vi "ZeroMQ_SUBGS.vi"() -> ()   [LabVIEW 2018]
uses:
  <vilib>/addons/zeromq/socket_type.ctl
  <vilib>/addons/zeromq/socket_options.ctl
  <vilib>/addons/zeromq/zeromq.lvlib
  <vilib>/addons/zeromq/zmq_socket.lvclass
  <vilib>/addons/zeromq/zmq_context.lvclass
panel:
  out "error out 5":errorcluster
  in  "stop 4":bool
  out "command 2":string
  out "reply":string
  out "message 2":string
  out "error out 4":errorcluster
  out "error out 3":errorcluster
  out "error out 2":errorcluster
  out "message":string
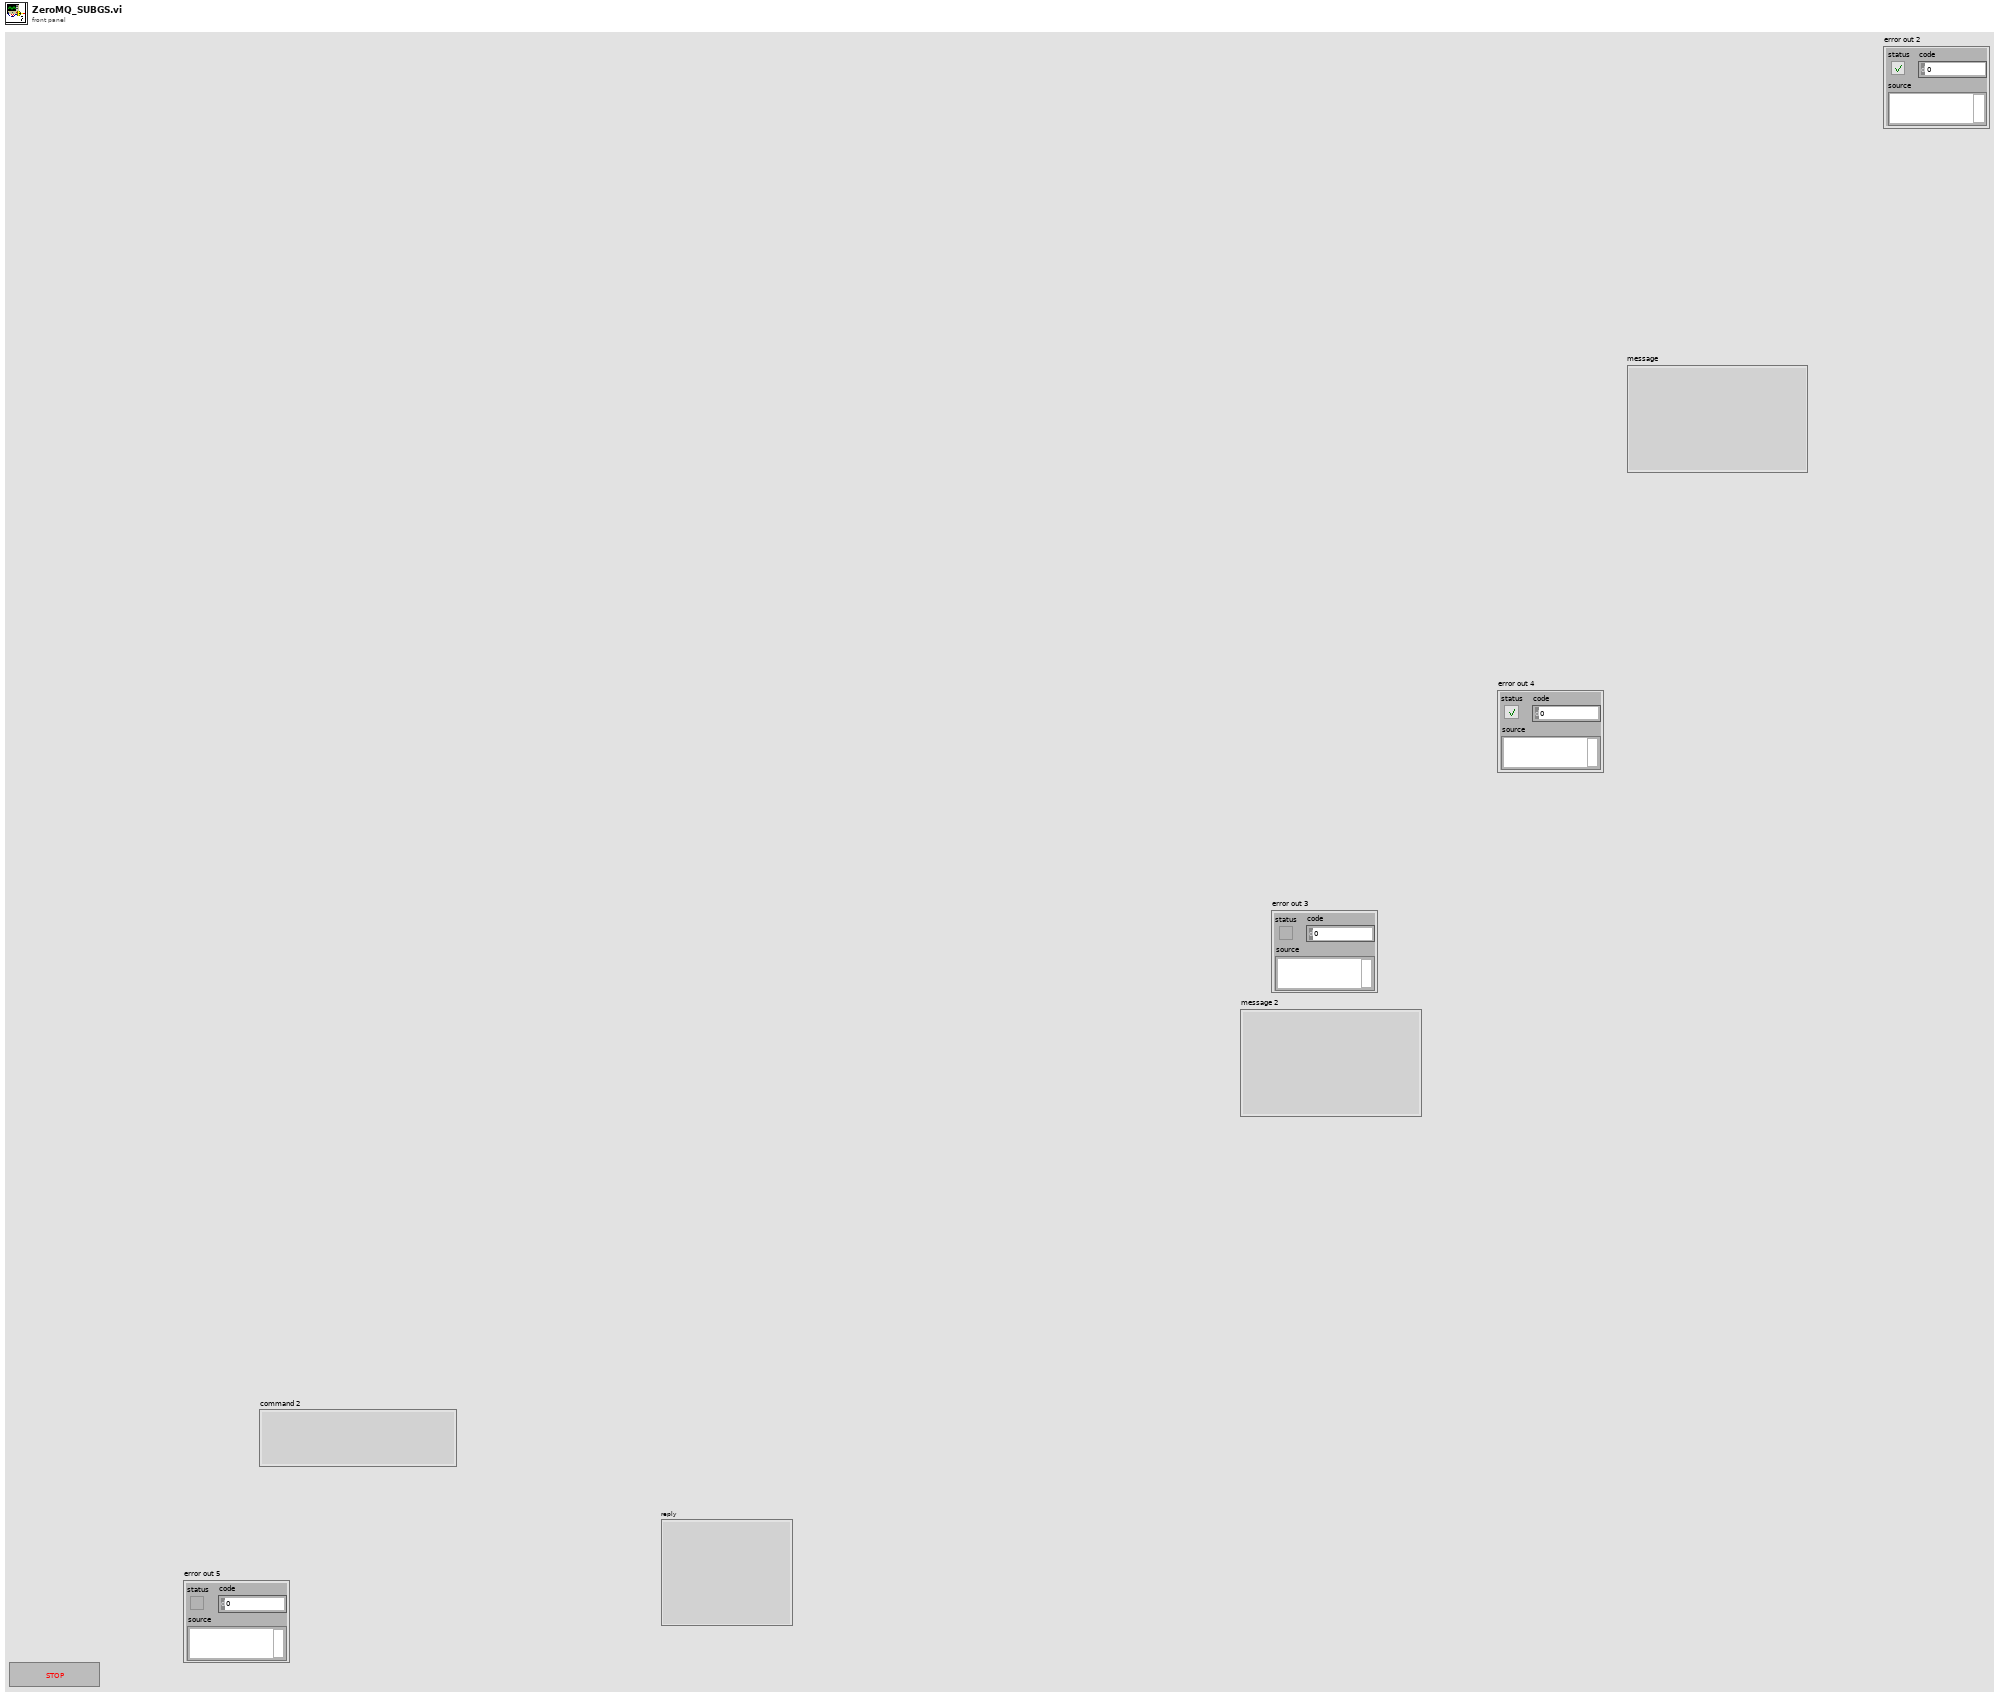
[diagram p1: front panel]
types:
  T1 = typedef "zeromq.lvlib/socket_options.ctl" = enum8{"NONE", "ZMQ_HWM", "<2>", "ZMQ_SWAP", "ZMQ_AFFINITY", "ZMQ_ROUTING_ID", "ZMQ_SUBSCRIBE", "ZMQ_UNSUBSCRIBE", "ZMQ_RATE", "ZMQ_RECOVERY_IVL", "ZMQ_MCAST_LOOP", "ZMQ_SNDBUF", "ZMQ_RCVBUF", "ZMQ_RCVMORE", "ZMQ_FD", "ZMQ_EVENTS", "ZMQ_TYPE", "ZMQ_LINGER", "ZMQ_RECONNECT_IVL", "ZMQ_BACKLOG", "ZMQ_RECOVERY_IVL_MSEC", "ZMQ_RECONNECT_IVL_MAX", "ZMQ_MAXMSGSIZE", "ZMQ_SNDHWM", "ZMQ_RCVHWM", "ZMQ_MULTICAST_HOPS", "<26>", "ZMQ_RCVTIMEO", "ZMQ_SNDTIMEO", "<29>", "<30>", "ZMQ_IPV4ONLY", "ZMQ_LAST_ENDPOINT", "ZMQ_ROUTER_MANDATORY", "ZMQ_TCP_KEEPALIVE", "ZMQ_TCP_KEEPALIVE_CNT", "ZMQ_TCP_KEEPALIVE_IDLE", "ZMQ_TCP_KEEPALIVE_INTVL", "ZMQ_TCP_ACCEPT_FILTER", "ZMQ_IMMEDIATE", "ZMQ_XPUB_VERBOSE", "ZMQ_ROUTER_RAW", "ZMQ_IPV6", "ZMQ_MECHANISM", "ZMQ_PLAIN_SERVER", "ZMQ_PLAIN_USERNAME", "ZMQ_PLAIN_PASSWORD", "ZMQ_CURVE_SERVER", "ZMQ_CURVE_PUBLICKEY", "ZMQ_CURVE_SECRETKEY", "ZMQ_CURVE_SERVERKEY", "ZMQ_PROBE_ROUTER", "ZMQ_REQ_CORRELATE", "ZMQ_REQ_RELAXED", "ZMQ_CONFLATE", "ZMQ_ZAP_DOMAIN", "ZMQ_ROUTER_HANDOVER", "ZMQ_TOS", "ZMQ_IPC_FILTER_PID", "ZMQ_IPC_FILTER_UID", "ZMQ_IPC_FILTER_GID", "ZMQ_CONNECT_ROUTING_ID", "ZMQ_GSSAPI_SERVER", "ZMQ_GSSAPI_PRINCIPAL", "ZMQ_GSSAPI_SERVICE_PRINCIPAL", "ZMQ_GSSAPI_PLAINTEXT", "ZMQ_HANDSHAKE_IVL", "<67>", "ZMQ_SOCKS_PROXY", "ZMQ_XPUB_NODROP", "ZMQ_BLOCKY", "ZMQ_XPUB_MANUAL", "ZMQ_XPUB_WELCOME_MSG", "ZMQ_STREAM_NOTIFY", "ZMQ_INVERT_MATCHING", "ZMQ_HEARTBEAT_IVL", "ZMQ_HEARTBEAT_TTL", "ZMQ_HEARTBEAT_TIMEOUT", "ZMQ_XPUB_VERBOSER", "ZMQ_CONNECT_TIMEOUT", "ZMQ_TCP_MAXRT", "ZMQ_THREAD_SAFE", "<82>", "<83>", "ZMQ_MULTICAST_MAXTPDU", "ZMQ_VMCI_BUFFER_SIZE", "ZMQ_VMCI_BUFFER_MIN_SIZE", "ZMQ_VMCI_BUFFER_MAX_SIZE", "ZMQ_VMCI_CONNECT_TIMEOUT", "ZMQ_USE_FD", "ZMQ_GSSAPI_PRINCIPAL_NAMETYPE", "ZMQ_GSSAPI_SERVICE_PRINCIPAL_NAMETYPE", "ZMQ_BINDTODEVICE", "ZMQ_ZAP_ENFORCE_DOMAIN", "ZMQ_LOOPBACK_FASTPATH", "ZMQ_METADATA", "ZMQ_MULTICAST_LOOP", "ZMQ_ROUTER_NOTIFY"}
  T2 = typedef "zeromq.lvlib/socket_type.ctl" = enum8{"ZMQ_PAIR", "ZMQ_PUB", "ZMQ_SUB", "ZMQ_REQ", "ZMQ_REP", "ZMQ_DEALER", "ZMQ_ROUTER", "ZMQ_PULL", "ZMQ_PUSH", "ZMQ_XPUB", "ZMQ_XSUB", "ZMQ_STREAM", "ZMQ_SERVER", "ZMQ_CLIENT", "ZMQ_RADIO", "ZMQ_DISH", "ZMQ_GATHER", "ZMQ_SCATTER", "ZMQ_DGRAM"}
  T3 = cluster{"ID":u32, "Address":string, "Service Name 1":string, "Service Name 2":string, "queue TX":refnum<queue>, "queue RX":refnum<queue>, "Port 1":u32, "Port 2":u32}
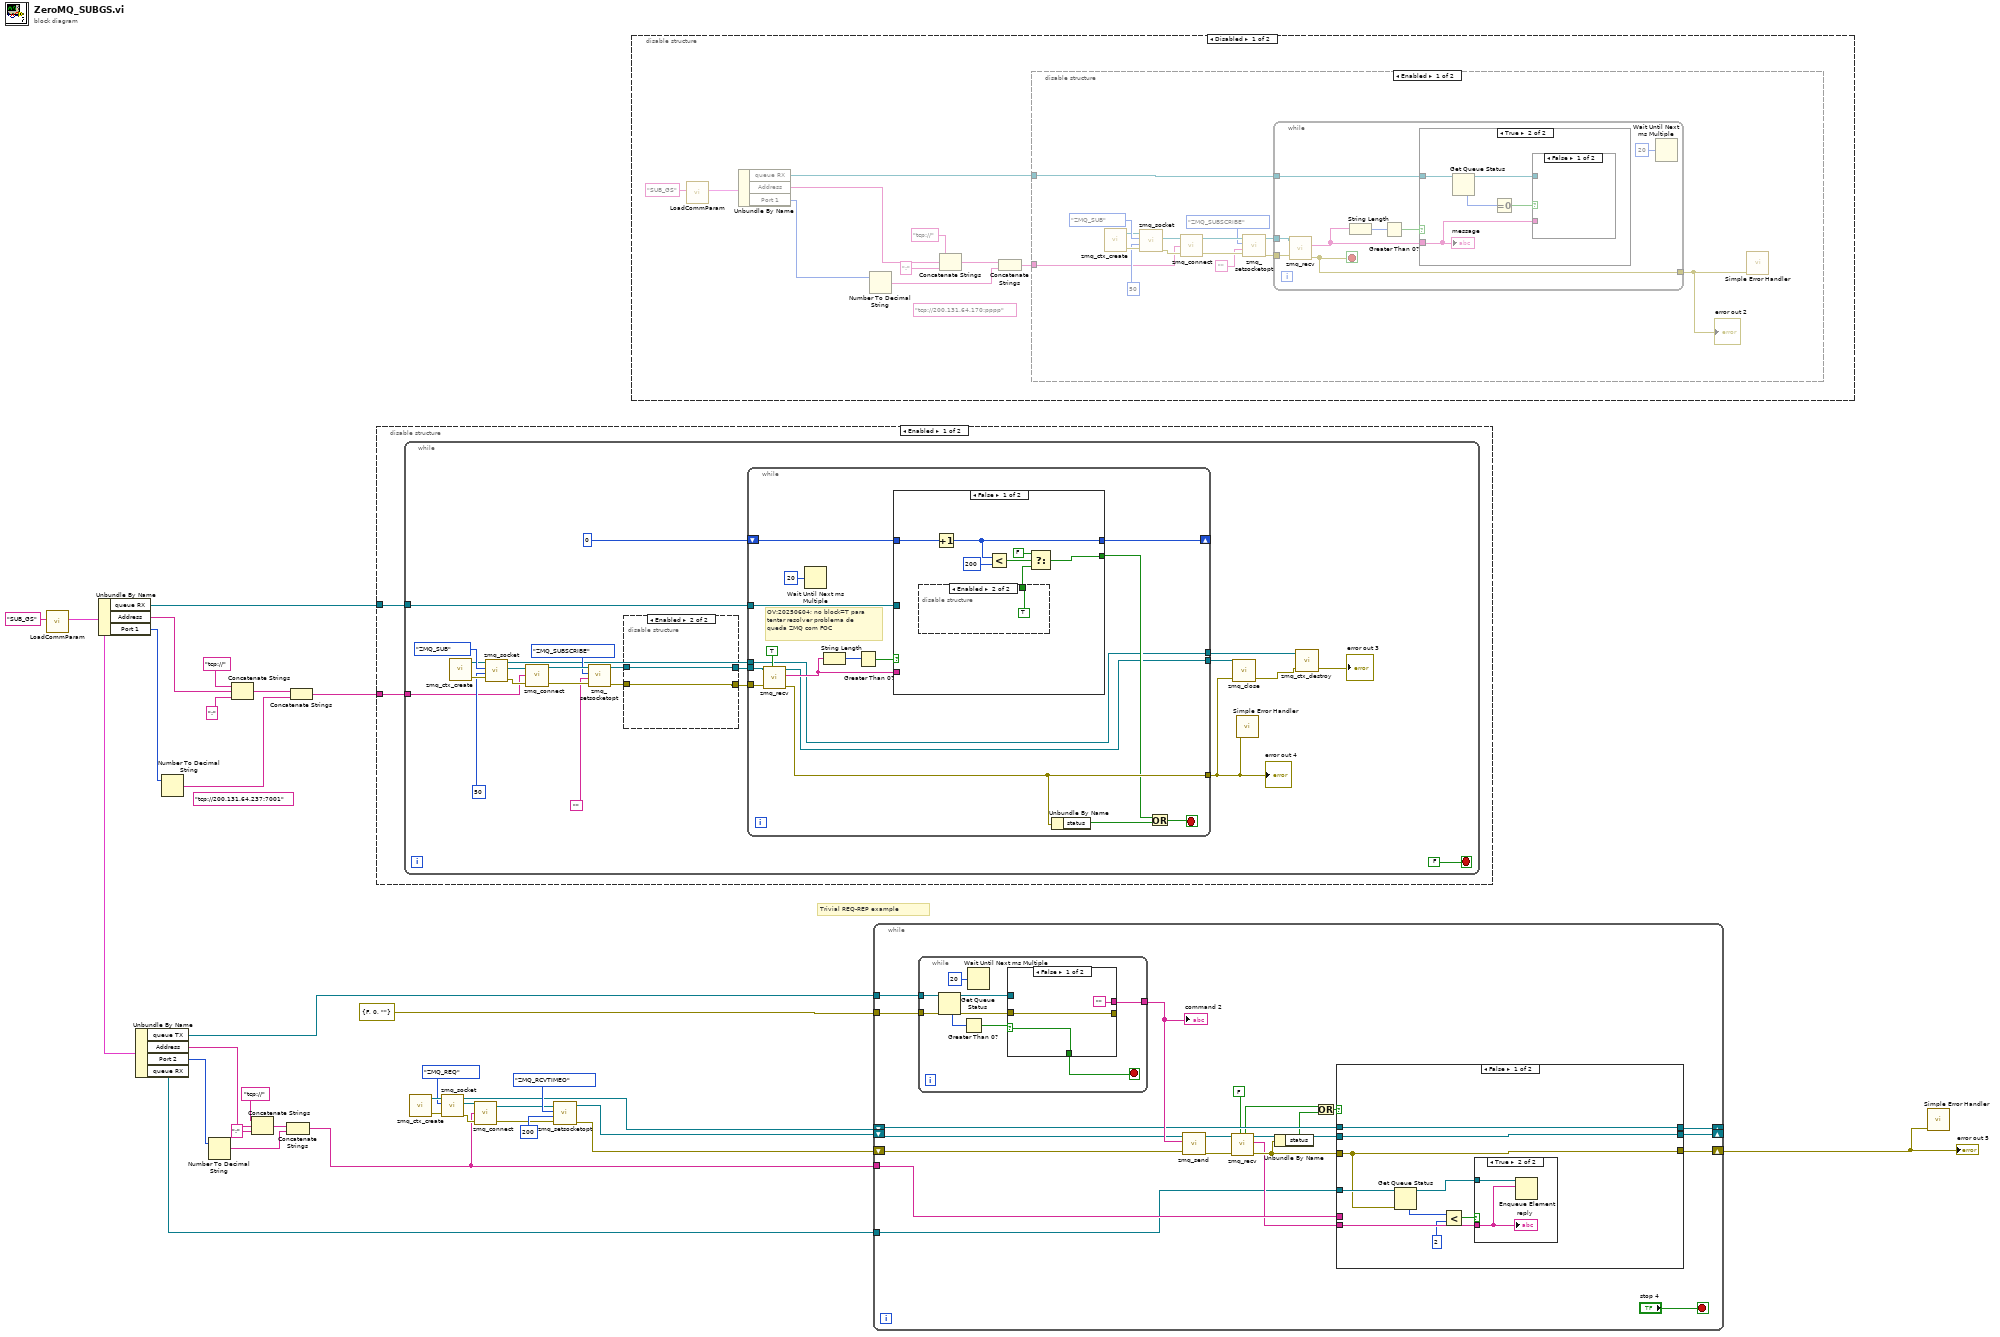
[diagram p0: block diagram]
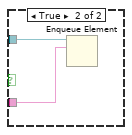
[diagram p3: hidden frame]
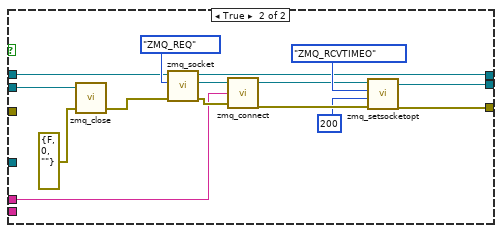
[diagram p7: hidden frame]
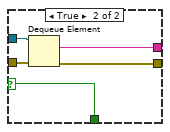
[diagram p8: hidden frame]
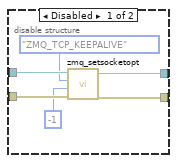
[diagram p9: hidden frame]
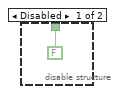
[diagram p10: hidden frame]
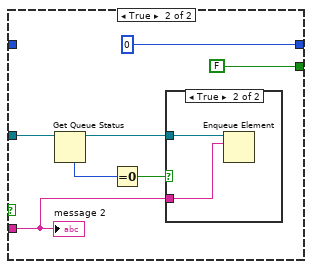
[diagram p11: hidden frame]
diagram:
  (unwired) "tcp://200.131.64.237:7001" ("endpoint")
  # "Trivial REQ-REP example"
  n1 = call "LoadCommParam.vi"("section name"="SUB_GS") -> ("output cluster"=w1:T3)  [unwired: 10 in]
  n2 = Unbundle By Name(w1) -> ("queue RX"=w25:refnum<queue>, "Address"=w32:string, "Port 1"=w31:u32)
  n3 = Unbundle By Name(w1) -> ("queue TX"=w16:refnum<queue>, "Address"=w18:string, "Port 2"=w17:u32, "queue RX"=w2:refnum<queue>)
  n4 = Number To Decimal String(number=w31) -> (decimal integer string=w30:string)  [unwired: 1 in]
  n5 = Number To Decimal String(number=w17) -> (decimal integer string=w22:string)  [unwired: 1 in]
  n6 = Concatenate Strings("tcp://" ("string"), w32, ":" ("string")) -> (w29:string)
  n7 = Concatenate Strings("tcp://" ("string"), w18, ":" ("string")) -> (w21:string)
  n8 = Concatenate Strings(w21, w22) -> (w10:string)
  n9 = Concatenate Strings(w29, w30) -> (w26:string)
  n10 = disable-structure shown="Enabled" {
    disable-tunnel: w25 -> [w35 _]
    disable-tunnel: w26 -> [w34 _]
    frame Enabled {
      n11 = while {
        tunnel: w35 -> [w50]
        tunnel: w34 -> [w49]
        stop <- FALSE stop-if-true
        n12 = call <vilib>:"zmq_ctx_create.vi"() -> ("error out"=w58:errorcluster, "context out"=w52:refnum<class "zmq_context.lvclass">)  [unwired: 4 in]
        n13 = call <vilib>:"zmq_socket.vi"("error in"=w58, "linger (ms)"=50, "socket type"=socket_type."ZMQ_SUB", "context in"=w52) -> ("error out"=w57:errorcluster, "socket out"=w53:refnum<class "zmq_socket.lvclass">, "context out"=w41:refnum<class "zmq_context.lvclass">)  [unwired: 1 in]
        n14 = call <vilib>:"zmq_connect.vi"("error in"=w57, "endpoint"=w49, "socket in"=w53) -> ("error out"=w55:errorcluster, "socket out"=w56:refnum<class "zmq_socket.lvclass">)  [unwired: 1 in]
        n15 = call <vilib>:"zmq_setsocketopt.vi"("error in"=w55, "value"="", "option"=socket_options."ZMQ_SUBSCRIBE", "socket in"=w56) -> ("error out"=w44:errorcluster, "socket out"=w46:refnum<class "zmq_socket.lvclass">)  [unwired: 2 in]
        n16 = disable-structure shown="Enabled" {
          disable-tunnel: w46 -> [w65 w67]
          disable-tunnel: [w64 w67] -> w45
          disable-tunnel: w44 -> [w63 w66]
          disable-tunnel: [w62 w66] -> w43
          frame Disabled {
            n17 = call <vilib>:"zmq_setsocketopt.vi"("error in"=w63, "value"=-1, "option"=socket_options."ZMQ_TCP_KEEPALIVE", "socket in"=w65) -> ("error out"=w62:errorcluster, "socket out"=w64:refnum<class "zmq_socket.lvclass">)  [unwired: 2 in]
          }
          frame Enabled {
          }
        }
        n18 = while {
          tunnel: w45 -> [w82]
          tunnel: w43 -> [w83]
          tunnel: [w73] -> w38
          tunnel: w50 -> [w79]
          shift-right: [w74] -> _
          shift-left: 0 -> [w75]
          tunnel: [w69] -> w40
          tunnel: w41 -> [w68]
          tunnel: [w68] -> w39
          stop <- w70 stop-if-true
          # "OV:20250604; no block=T para\ntentar resolver problema de\nqueda ZMQ com FOC"
          n19 = call <vilib>:"zmq_recv.vi"("no block? (F)"=TRUE, "error in"=w83, "socket in"=w82) -> ("error out"=w73:errorcluster, "data"=w78:string, "socket out"=w69:refnum<class "zmq_socket.lvclass">)  [unwired: 2 in, 2 out]
          n20 = Wait Until Next ms Multiple(millisecond multiple=u32 20) -> ()  [unwired: 1 out]
          n21 = String Length(string=w78) -> (length=w81:i32)
          n22 = Greater Than 0?(x=w81) -> (x > 0?=w80:bool)
          n23 = case shown="False" w80 {
            tunnel: w79 -> [_ w98]
            tunnel: w78 -> [_ w95]
            tunnel: w75 -> [w90 _]
            tunnel: [w89 0] -> w74
            tunnel: [w86 FALSE] -> w71
            frame False {
              n24 = disable-structure shown="Enabled" {
                disable-tunnel: [FALSE ("f") TRUE] -> w84
                frame Disabled {
                }
                frame Enabled {
                }
              }
              n25 = Increment(x=w90) -> (x+1=w89:i32)
              n26 = Less?(x=w89, y=200) -> (x < y?=w87:bool)
              n27 = Select(t=FALSE, s=w87, f=w84) -> (s? t:f=w86:bool)
            }
            frame True {
              n28 = Get Queue Status(queue=w98) -> (queue out=w96:refnum<queue>, # elements in queue=w99:i32)  [unwired: 2 in, 6 out]
              n29 = Equal To 0?(x=w99) -> (x = 0?=w97:bool)
              n30 = case shown="True" w97 {
                tunnel: w96 -> [_ w101]
                tunnel: w95 -> [_ w100]
                frame False {
                }
                frame True {
                  n31 = Enqueue Element(queue=w101, element=w100) -> ()  [unwired: 2 in, 3 out]
                }
              }
              "message 2" <- w95
            }
          }
          n32 = Unbundle By Name(w73) -> ("status"=w72:bool)
          n33 = Or(x=w71, y=w72) -> (x .or. y?=w70:bool)
        }
        "error out 4" <- w38
        n34 = call <vilib>:"zmq_close.vi"("error in"=w38, "socket"=w40) -> ("error out"=w37:errorcluster)  [unwired: 3 in]
        n35 = call <vilib>:"Simple Error Handler.vi"("error in (no error)"=w38) -> ()  [unwired: 4 in, 5 out]
        n36 = call <vilib>:"zmq_ctx_destroy.vi"("error in"=w37, "context in"=w39) -> ("error out"=→"error out 3":errorcluster)  [unwired: 3 in]
      }
    }
    frame Disabled {
    }
  }
  n37 = call <vilib>:"zmq_ctx_create.vi"() -> ("error out"=w15:errorcluster, "context out"=w12:refnum<class "zmq_context.lvclass">)  [unwired: 4 in]
  n38 = call <vilib>:"zmq_socket.vi"("error in"=w15, "socket type"=socket_type."ZMQ_REQ", "context in"=w12) -> ("error out"=w13:errorcluster, "socket out"=w14:refnum<class "zmq_socket.lvclass">, "context out"=w5:refnum<class "zmq_context.lvclass">)  [unwired: 2 in]
  n39 = call <vilib>:"zmq_connect.vi"("error in"=w13, "endpoint"=w10, "socket in"=w14) -> ("error out"=w6:errorcluster, "socket out"=w7:refnum<class "zmq_socket.lvclass">)  [unwired: 1 in]
  n40 = call <vilib>:"zmq_setsocketopt.vi"("error in"=w6, "value"=200 ("max queue size (-1, unlimited)"), "option"=socket_options."ZMQ_RCVTIMEO", "socket in"=w7) -> ("error out"=w3:errorcluster, "socket out"=w4:refnum<class "zmq_socket.lvclass">)  [unwired: 2 in]
  n41 = disable-structure shown="Disabled" {
    frame Disabled {
      (unwired) "tcp://200.131.64.170:pppp" ("endpoint")
      n42 = call "LoadCommParam.vi"("section name"="SUB_GS") -> ("output cluster"=w102:T3)  [unwired: 10 in]
      n43 = Unbundle By Name(w102) -> ("queue RX"=w103:refnum<queue>, "Address"=w110:string, "Port 1"=w109:u32)
      n44 = Number To Decimal String(number=w109) -> (decimal integer string=w108:string)  [unwired: 1 in]
      n45 = Concatenate Strings("tcp://" ("string"), w110, ":" ("string")) -> (w107:string)
      n46 = Concatenate Strings(w107, w108) -> (w104:string)
      n47 = disable-structure shown="Enabled" {
        disable-tunnel: w103 -> [w113 _]
        disable-tunnel: w104 -> [w112 _]
        frame Enabled {
          n48 = call <vilib>:"zmq_ctx_create.vi"() -> ("error out"=w125:errorcluster, "context out"=w115:refnum<class "zmq_context.lvclass">)  [unwired: 4 in]
          n49 = call <vilib>:"zmq_socket.vi"("error in"=w125, "linger (ms)"=50, "socket type"=socket_type."ZMQ_SUB", "context in"=w115) -> ("error out"=w124:errorcluster, "socket out"=w116:refnum<class "zmq_socket.lvclass">)  [unwired: 1 in, 1 out]
          n50 = call <vilib>:"zmq_connect.vi"("error in"=w124, "endpoint"=w112, "socket in"=w116) -> ("error out"=w122:errorcluster, "socket out"=w123:refnum<class "zmq_socket.lvclass">)  [unwired: 1 in]
          n51 = call <vilib>:"zmq_setsocketopt.vi"("error in"=w122, "value"="", "option"=socket_options."ZMQ_SUBSCRIBE", "socket in"=w123) -> ("error out"=w121:errorcluster, "socket out"=w120:refnum<class "zmq_socket.lvclass">)  [unwired: 2 in]
          n52 = while {
            tunnel: w120 -> [w132]
            tunnel: w121 -> [w134]
            tunnel: [w133] -> w117
            tunnel: w113 -> [w129]
            stop <- w133 stop-if-true
            n53 = call <vilib>:"zmq_recv.vi"("error in"=w134, "socket in"=w132) -> ("error out"=w133:errorcluster, "data"=w128:string)  [unwired: 3 in, 3 out]
            n54 = String Length(string=w128) -> (length=w131:i32)
            n55 = Greater Than 0?(x=w131) -> (x > 0?=w130:bool)
            n56 = case shown="True" w130 {
              tunnel: w129 -> [_ w138]
              tunnel: w128 -> [_ w135]
              frame False {
              }
              frame True {
                n57 = Get Queue Status(queue=w138) -> (queue out=w136:refnum<queue>, # elements in queue=w139:i32)  [unwired: 2 in, 6 out]
                n58 = Equal To 0?(x=w139) -> (x = 0?=w137:bool)
                n59 = case shown="False" w137 {
                  tunnel: w136 -> [_ w141]
                  tunnel: w135 -> [_ w140]
                  frame False {
                  }
                  frame True {
                    n60 = Enqueue Element(queue=w141, element=w140) -> ()  [unwired: 2 in, 3 out]
                  }
                }
                "message" <- w135
              }
            }
            n61 = Wait Until Next ms Multiple(millisecond multiple=u32 20) -> ()  [unwired: 1 out]
          }
          "error out 2" <- w117
          n62 = call <vilib>:"Simple Error Handler.vi"("error in (no error)"=w117) -> ()  [unwired: 4 in, 5 out]
        }
        frame Disabled {
        }
      }
    }
    frame Enabled {
    }
  }
  n63 = while {
    tunnel: w16 -> [w162]
    tunnel: errorcluster {"status"=FALSE, "code"=0, "source"=""} ("error out") -> [w158]
    tunnel: w10 -> [w147]
    shift-right: [w146] -> _
    shift-left: w5 -> [w157]
    shift-right: [w145] -> _
    shift-left: w4 -> [w156]
    shift-right: [w159] -> w24
    shift-left: w3 -> [w144]
    tunnel: w2 -> [w142]
    stop <- "stop 4" stop-if-true
    n64 = while {
      tunnel: w162 -> [w196]
      tunnel: w158 -> [w195]
      tunnel: [w191] -> w161
      stop <- w190 stop-if-true
      n65 = Get Queue Status(queue=w196, error in (no error)=w195) -> (queue out=w192:refnum<queue>, error out=w193:errorcluster, # elements in queue=w197:i32)  [unwired: 1 in, 5 out]
      n66 = Greater Than 0?(x=w197) -> (x > 0?=w194:bool)
      n67 = Wait Until Next ms Multiple(millisecond multiple=u32 20) -> ()  [unwired: 1 out]
      n68 = case shown="False" w194 {
        selector: w194 -> [w198 w201]
        tunnel: w193 -> [w200 w205]
        tunnel: w192 -> [_ w204]
        tunnel: [w200 w203] -> _
        tunnel: ["" w202] -> w191
        tunnel: [w198 w201] -> w190
        frame False {
        }
        frame True {
          n69 = Dequeue Element(queue=w204, error in (no error)=w205) -> (element=w202:string, error out=w203:errorcluster)  [unwired: 1 in, 2 out]
        }
      }
    }
    "command 2" <- w161
    n70 = call <vilib>:"zmq_send.vi"("error in"=w144, "data"=w161, "socket in"=w156) -> ("error out"=w154:errorcluster, "socket out"=w155:refnum<class "zmq_socket.lvclass">)  [unwired: 4 in]
    n71 = call <vilib>:"zmq_recv.vi"("no block? (F)"=FALSE, "error in"=w154, "socket in"=w155) -> ("error out"=w149:errorcluster, "data"=w143:string, "socket out"=w148:refnum<class "zmq_socket.lvclass">, "timeout?"=w150:bool)  [unwired: 2 in, 1 out]
    n72 = Unbundle By Name(w149) -> ("status"=w151:bool)
    n73 = Or(x=w150, y=w151) -> (x .or. y?=w152:bool)
    n74 = case shown="False" w152 {
      tunnel: [w166 w176] -> w159
      tunnel: w157 -> [w170 w178]
      tunnel: w149 -> [w166 _]
      tunnel: w148 -> [w171 w179]
      tunnel: w147 -> [_ w177]
      tunnel: [w171 w175] -> w145
      tunnel: [w170 w174] -> w146
      tunnel: w143 -> [w168 _]
      tunnel: w142 -> [w167 _]
      frame False {
        n75 = Get Queue Status(queue=w167, error in (no error)=w166) -> (queue out=w169:refnum<queue>, # elements in queue=w164:i32)  [unwired: 1 in, 6 out]
        n76 = Less?(x=w164, y=2) -> (x < y?=w165:bool)
        n77 = case shown="True" w165 {
          tunnel: w169 -> [_ w173]
          tunnel: w168 -> [_ w172]
          frame False {
          }
          frame True {
            n78 = Enqueue Element(queue=w173, element=w172) -> ()  [unwired: 2 in, 3 out]
            "reply" <- w172
          }
        }
      }
      frame True {
        n79 = call <vilib>:"zmq_close.vi"("error in"=errorcluster {"status"=FALSE, "code"=0, "source"=""}, "socket"=w179) -> ("error out"=w181:errorcluster)  [unwired: 3 in]
        n80 = call <vilib>:"zmq_socket.vi"("error in"=w181, "socket type"=socket_type."ZMQ_REQ", "context in"=w178) -> ("error out"=w187:errorcluster, "socket out"=w188:refnum<class "zmq_socket.lvclass">, "context out"=w174:refnum<class "zmq_context.lvclass">)  [unwired: 2 in]
        n81 = call <vilib>:"zmq_connect.vi"("error in"=w187, "endpoint"=w177, "socket in"=w188) -> ("error out"=w183:errorcluster, "socket out"=w184:refnum<class "zmq_socket.lvclass">)  [unwired: 1 in]
        n82 = call <vilib>:"zmq_setsocketopt.vi"("error in"=w183, "value"=200 ("max queue size (-1, unlimited)"), "option"=socket_options."ZMQ_RCVTIMEO", "socket in"=w184) -> ("error out"=w176:errorcluster, "socket out"=w175:refnum<class "zmq_socket.lvclass">)  [unwired: 2 in]
      }
    }
  }
  "error out 5" <- w24
  n83 = call <vilib>:"Simple Error Handler.vi"("error in (no error)"=w24) -> ()  [unwired: 4 in, 5 out]
